vi "CrossDispense.vi"(4 "speed_uL_s":dbl, 5 "wasteLine":string, 6 "drawVolume_ul":dbl, 7 "airWaste2":string, 9 "dispenseLine":string, 10 "drawAnalyte":string, 11 "Pump in":refnum<k24>) -> (0 "Pump out":refnum<k24>, 3 "log":string)   [LabVIEW 2020]
uses:
  D:/PumpAutomation2/DEMPBot2/PumpAdapter.exe
  PumpAdapter.exe
panel:
  out "Draw":string
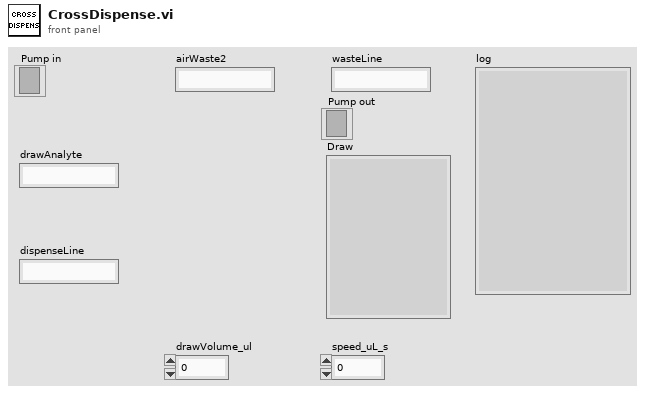
[diagram p1: front panel]
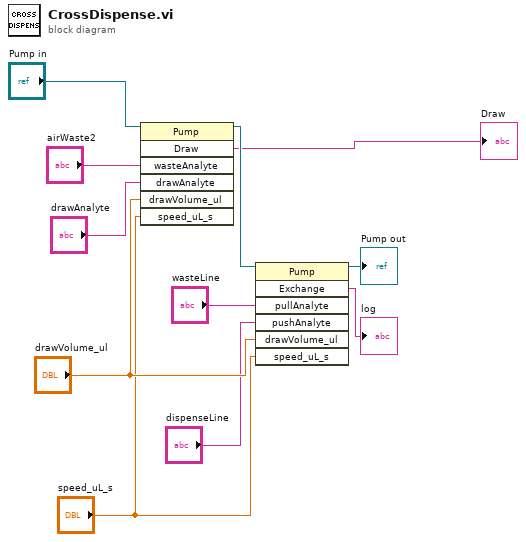
[diagram p0: block diagram]
diagram:
  n1 = invoke class="Pump" method="Draw"(reference="Pump in", "wasteAnalyte"="airWaste2", "drawAnalyte"="drawAnalyte", "drawVolume_ul"="drawVolume_ul", "speed_uL_s"="speed_uL_s") -> (reference out=w4:refnum<k24>, "Draw"=→"Draw":string)  [unwired: 2 in, 5 out]
  n2 = invoke class="Pump" method="Exchange"(reference=w4, "pullAnalyte"="wasteLine", "pushAnalyte"="dispenseLine", "drawVolume_ul"="drawVolume_ul", "speed_uL_s"="speed_uL_s") -> (reference out=→"Pump out":refnum<k24>, "Exchange"=→"log":string)  [unwired: 2 in, 5 out]
